vi "SONG.vi"() -> ()   [LabVIEW 2017]
panel:
  out "SONG":string
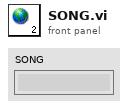
[diagram p1: front panel]
diagram:
